vi "collision.vi"(4 "error in":errorcluster={"status"=FALSE, "code"=0, "source"="Event Code: 0\r\ncomplete\r\n-----------------------------------\nEvent Code: 0\r\nweather configured to \"Default\"\r\n-----------------------------------\nEvent Code: 0\r\n\r\n-----------------------------------\n"}, 7 "Collision sensor configuration":string=" {\n    \"type\": \"Collision\",\n    \"listen_port\": 8800,\n    \"debug_drawing\": false,\n    \"desired_tags\": [\n      \"vt\"\n    ],\n  \"undesired_tags\": [\n  \"static\"\n  ]\n}") -> (0 "error out":errorcluster={"status"=FALSE, "code"=0, "source"="Event Code: 0\r\ncomplete\r\n-----------------------------------\nEvent Code: 0\r\nweather configured to \"Default\"\r\n-----------------------------------\nEvent Code: 0\r\n\r\n-----------------------------------\n"}, 1 "Collision sensor configuration":string="[\n {\n    \"type\": \"Collision\",\n    \"listen_port\": 8800,\n    \"packet_size\": 1472,\n    \"debug_drawing\": true,\n    \"desired_tags\": [\n      \"vt\"\n    ],\n  \"undesired_tags\": [\n  \"static\"\n  ]\n}\n\n]", 2 "Accumulative sensor sample":string[](array[string]), 3 "Collision sensor sample":string)   [LabVIEW 2019]
doc: "Configure and sample the Collision sensor. Outputs information on the Time to collision, among other relevant information to detect a collision with vehicles or objects with the tag \"vt\""
uses:
  controls/Header.ctl
  tools/simx_common.vi
panel:
  out "Header":T1 {"game_time" format="%_10g"}
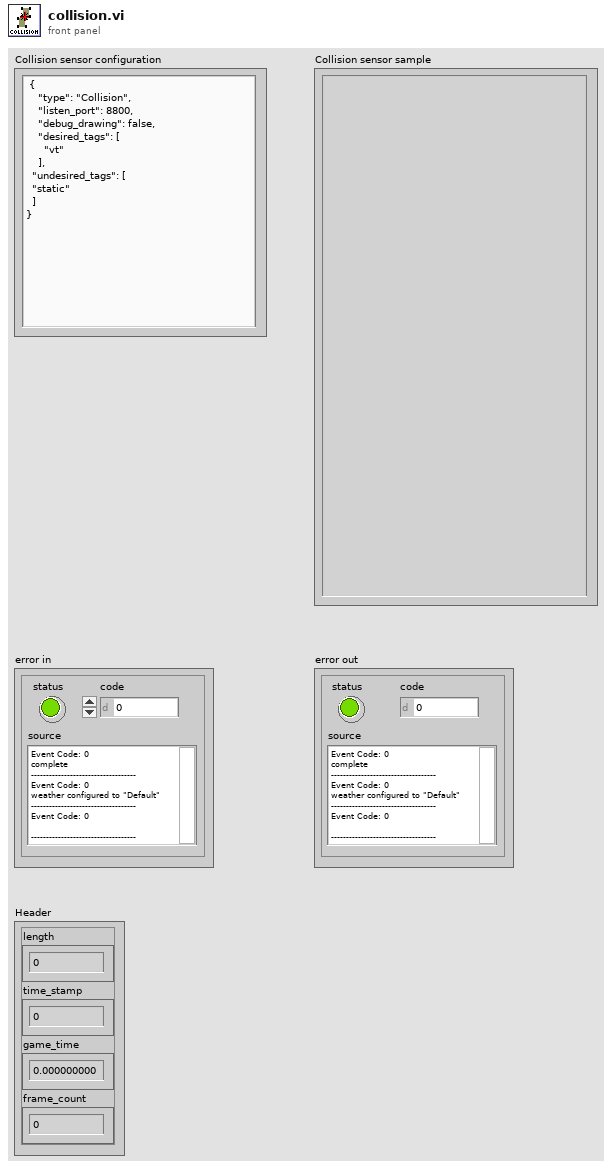
[diagram p1: front panel]
types:
  T1 = typedef "Header.ctl" = cluster{"length":u32, "time_stamp":u32, "game_time":sgl, "frame_count":u32}
  T2 = typedef "simx_connection.ctl" = cluster{"Config":T3, "Connections":T6, "Map":cluster{"lanes":cluster{"x":dbl[], "y":dbl[], "z":dbl[]}, "StartPosition":cluster{"start_points":T7, "StartRotation":dbl[], "StartLocation":dbl[]}, "Draw Map Size":T8, "DrawArea":cluster{"min_Y":dbl, "min_X":dbl, "Scale X":dbl, "Scale Y":dbl}, "Map":picture, "Map Geojson":string}}
  T3 = typedef "config.ctl" = cluster{"Trajectory":T4, "Weather":T5}
  T4 = typedef "trajectory.ctl" = cluster{"Number of frames":i32, "Frame number":i32, "Trajectory":string}
  T5 = typedef "weather.ctl" = cluster{"id":string}
  T6 = typedef "connections.ctl" = cluster{"Simulator Connection":refnum<k5>, "server_ip":string, "Port":i32, "Sensor connections":refnum<k5>[]}
  T7 = typedef "start_points.ctl" = cluster{"locations":dbl[][], "rotations":dbl[][], "type":string[]}
  T8 = typedef "LVBoundsTypeDef.ctl" = cluster{"Width":u32, "Height":u32}
  T9 = typedef "sensor_sample.ctl" = cluster{"Header":T1, "data out":string}
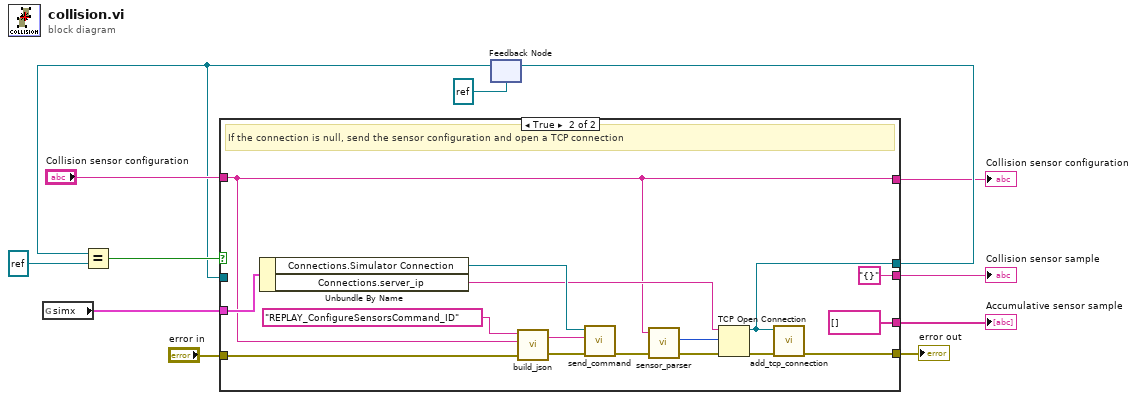
[diagram p0: block diagram]
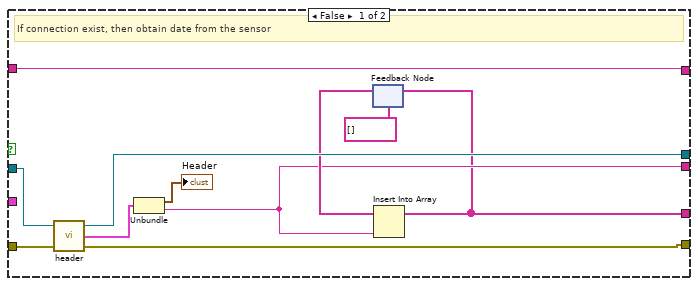
[diagram p2: hidden frame]
diagram:
  n1 = global read "simx_common.vi" "simx"() -> (w1:T2)
  n2 = feedback #1(refnum<k5> refnum ("state_connection")) -> (w6:refnum<k5>)
  n3 = Equal?(x=w6, y=refnum<k5> refnum ("null connection")) -> (x = y?=w8:bool)
  n4 = case shown="True" w8 {
    tunnel: [w19 w25] -> w12
    tunnel: "Collision sensor configuration" -> [w20 w27]
    tunnel: [w18 w24] -> w9
    tunnel: w6 -> [w23 _]
    tunnel: "error in" -> [w22 w33]
    tunnel: [w16 "{}" ("data out")] -> w5
    tunnel: [w20 w27] -> w4
    tunnel: [w15 string[] []] -> w2
    tunnel: w1 -> [_ w31]
    frame False {
      # "If connection exist, then obtain date from the sensor"
      n5 = call "header.vi"("error in"=w22, "TCP Network Connection in"=w23) -> ("error out"=w19:errorcluster, "Sensor sample"=w21:T9, "TCP Network Connection out"=w18:refnum<k5>)  [unwired: 1 in]
      n6 = Unbundle(w21) -> ("Header"=→"Header":T1, "data out"=w16:string)
      n7 = feedback #2(string[] []) -> (w17:string[])
      n8 = Insert Into Array(array=w17, new element=w16) -> (w15:string[])  [unwired: 1 in]
      n9 = feedback-in #2(w15) -> ()
    }
    frame True {
      # "If the connection is null, send the sensor configuration and open a TCP connection"
      n10 = Unbundle By Name(w31) -> ("Connections.Simulator Connection"=w30:refnum<k5>, "Connections.server_ip"=w29:string)
      n11 = call "build_json.vi"("error in"=w33, "Message"=w27, "Command_ID"="REPLAY_ConfigureSensorsCommand_ID") -> ("error out"=w37:errorcluster, "JSON Out"=w38:string)  [unwired: 1 in]
      n12 = call "send_command.vi"("error in"=w37, "JSON Command"=w38, "TCP Network Connection in"=w30) -> ("error out"=w36:errorcluster)  [unwired: 1 in, 3 out]
      n13 = call "sensor_parser.vi"("Sensor configuration"=w27, "error in"=w36) -> ("Port out"=w26:u16, "error out"=w28:errorcluster)  [unwired: 1 in, 2 out]
      n14 = TCP Open Connection(address=w29, remote port or service name=w26, error in (no error)=w28) -> (connection ID=w24:refnum<k5>, error out=w35:errorcluster)  [unwired: 2 in]
      n15 = call "add_tcp_connection.vi"("error in"=w35, "Sensor connection"=w24) -> ("error out"=w25:errorcluster)  [unwired: 5 in]
    }
  }
  "error out" <- w12
  "Collision sensor sample" <- w5
  "Collision sensor configuration" <- w4
  "Accumulative sensor sample" <- w2
  n16 = feedback-in #1(w9) -> ()
